vi "solar_qtimer Set.vi"(6 "Suppress Errors? (T)":bool=TRUE, 7 "Target Name":string, 8 "error in (no error)":errorcluster, 10 "Settings":T1={"QTimer"="", "Delay"=0, "Start"=FALSE, "EnQ_Type"=enum."IgnoreIfExists", "Messages"=[]}, 11 "QTimer Refnum in":T2) -> (0 "error out":errorcluster, 3 "QTimer Refnum out":T2)   [LabVIEW 2018]
doc: "This sets the start/stop of the QTimer by name."
uses:
  solar_qtimer_ctl Refnum.ctl
  solar_qtimer_ctl QTimer Settings.ctl
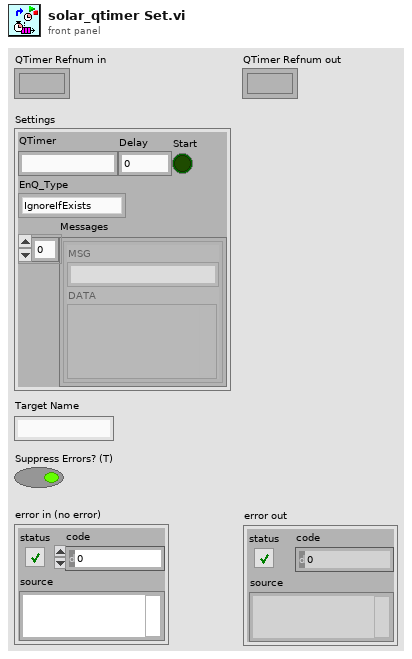
[diagram p1: front panel]
types:
  T1 = typedef "solar_qtimer_ctl QTimer Settings.ctl" = cluster{"QTimer":string, "Delay":i32, "Start":bool, "EnQ_Type":enum8{"Normal", "Priority", "IgnoreIfExists"}, "Messages":cluster{"MSG":string, "DATA":variant}[]}
  T2 = typedef "solar_qtimer_ctl Refnum.ctl" = refnum<k1>
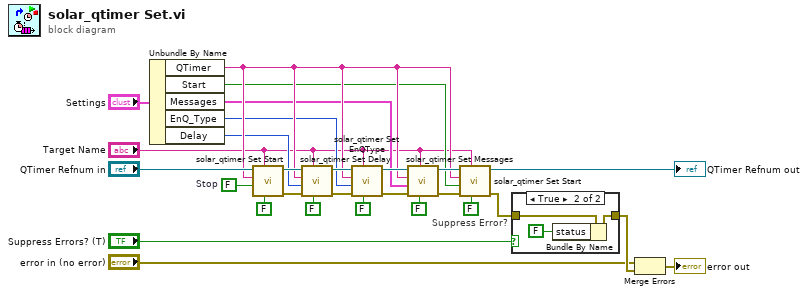
[diagram p0: block diagram]
diagram:
  w8 = FALSE  # Stop
  n1 = Unbundle By Name("Settings") -> ("QTimer"=w6:string, "Start"=w4:bool, "Messages"=w3:cluster{"MSG":string, "DATA":variant}[], "EnQ_Type"=w2:enum8{"Normal", "Priority", "IgnoreIfExists"}, "Delay"=w5:i32)
  n2 = call "solar_qtimer Set Start.vi"("Suppress Errors? (T)"=FALSE, "Target Name"="Target Name", "Start (F = Stop)"=w8, "QTimer Name"=w6, "QTimer Refnum in"="QTimer Refnum in") -> ("error out"=w9:errorcluster, "QTimer Refnum out"=w10:T2)  [unwired: 5 in]
  n3 = call "solar_qtimer Set Delay.vi"("Suppress Errors? (T)"=FALSE, "Target Name"="Target Name", "error in (no error)"=w9, "Delay (-1)"=w5, "QTimer Name"=w6, "QTimer Refnum in"=w10) -> ("error out"=w23:errorcluster, "QTimer Refnum out"=w24:T2)  [unwired: 4 in]
  n4 = call "solar_qtimer Set EnQType.vi"("Suppress Errors? (T)"=FALSE, "Target Name"="Target Name", "error in (no error)"=w23, "EnQ_Type (IgnoreIfExists)"=w2, "QTimer Name"=w6, "QTimer Refnum in"=w24) -> ("error out"=w22:errorcluster, "QTimer Refnum out"=w21:T2)  [unwired: 4 in]
  n5 = call "solar_qtimer Set Messages.vi"("Suppress Errors? (T)"=FALSE, "Target Name"="Target Name", "error in (no error)"=w22, "Messages"=w3, "QTimer Name"=w6, "QTimer Refnum in"=w21) -> ("error out"=w15:errorcluster, "QTimer Refnum out"=w17:T2)  [unwired: 4 in]
  n6 = call "solar_qtimer Set Start.vi"("Suppress Errors? (T)"=FALSE, "Target Name"="Target Name", "error in (no error)"=w15, "Start (F = Stop)"=w4, "QTimer Name"=w6, "QTimer Refnum in"=w17) -> ("error out"=w14:errorcluster, "QTimer Refnum out"=→"QTimer Refnum out":T2)  [unwired: 4 in]
  n7 = case "Suppress Error?" shown="True" "Suppress Errors? (T)" {
    tunnel: w14 -> [w29 w32]
    tunnel: [w29 w31] -> w27
    frame False {
    }
    frame True {
      n8 = Bundle By Name(cluster=w32, "status"=FALSE) -> (w31:errorcluster)
    }
  }
  n9 = Merge Errors("error in (no error)", w27) -> (→"error out":errorcluster)
